vi "Statemachine.vi"() -> ()   [LabVIEW 2017]
uses:
  State machin control.ctl
panel:
  in  "State":T1
  out "Current State":enum16{"Start", "State 1", "State 2", "Stop"}(ring)
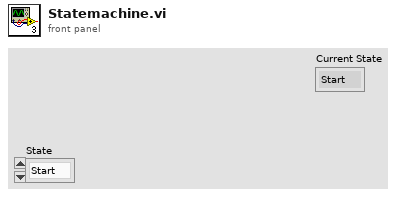
[diagram p1: front panel]
types:
  T1 = typedef "State machin control.ctl" = enum16{"Start", "State 1", "State 2", "Stop"}
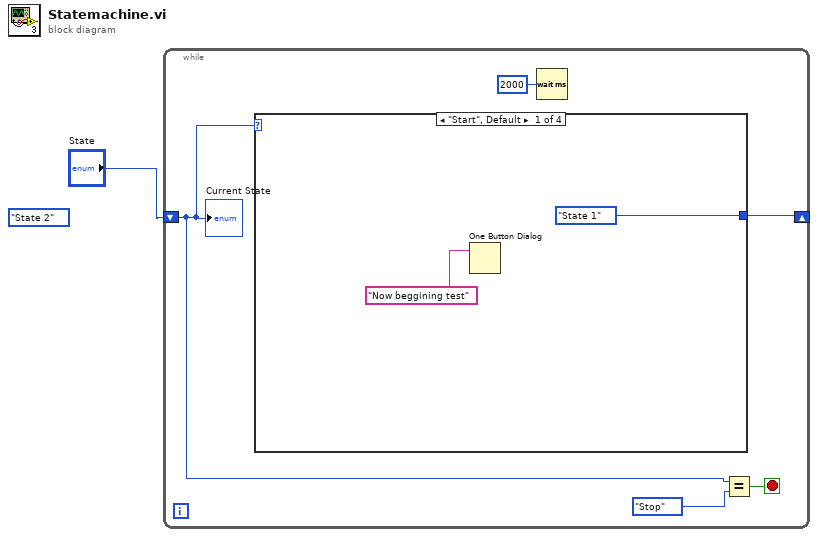
[diagram p0: block diagram]
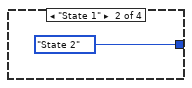
[diagram p2: hidden frame]
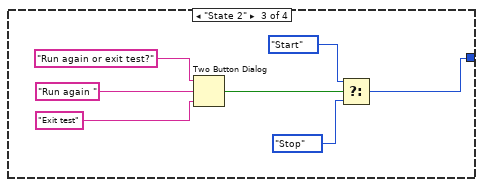
[diagram p3: hidden frame]
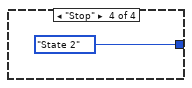
[diagram p4: hidden frame]
diagram:
  (unwired) enum16{"Start", "State 1", "State 2", "Stop"}."State 2"
  n1 = while {
    shift-right: [w6] -> _
    shift-left: "State" -> [w3]
    stop <- w4 stop-if-true
    n2 = case shown="\"Start\", Default" w3 {
      tunnel: [enum16{"Start", "State 1", "State 2", "Stop"}."State 1" enum16{"Start", "State 1", "State 2", "Stop"}."State 2" w15 enum16{"Start", "State 1", "State 2", "Stop"}."State 2"] -> w6
      frame "Start", Default {
        n3 = One Button Dialog(message="Now beggining test") -> ()  [unwired: 1 in, 1 out]
      }
      frame "State 1" {
      }
      frame "State 2" {
        n4 = Two Button Dialog(message="Run again or exit test?", 1:"Exit test", 2:"Run again ") -> (T button?=w10:bool)
        n5 = Select(t=enum16{"Start", "State 1", "State 2", "Stop"}."Start", s=w10, f=enum16{"Start", "State 1", "State 2", "Stop"}."Stop") -> (s? t:f=w15:enum16{"Start", "State 1", "State 2", "Stop"})
      }
      frame "Stop" {
      }
    }
    n6 = Wait (ms)(milliseconds to wait=u32 2000) -> ()  [unwired: 1 out]
    n7 = Equal?(x=w3, y=enum16{"Start", "State 1", "State 2", "Stop"}."Stop") -> (x = y?=w4:bool)
    "Current State" <- w3
  }
